vi "Threshold (subVI).vi"(8 "error in (no error)":errorcluster, 11 "Image  in":T1=refnum) -> (0 "error out":errorcluster, 2 "Cluster":cluster{sgl, "element":sgl}, 3 "Histogram":T2(graph))   [LabVIEW 2013]
uses:
  <vilib>/vision/Image Controls.llb/IMAQ Image.ctl
  <vilib>/vision/NI_Vision_Development_Module.lvlib
panel:
  out "brightened image":T1(plugin-control)
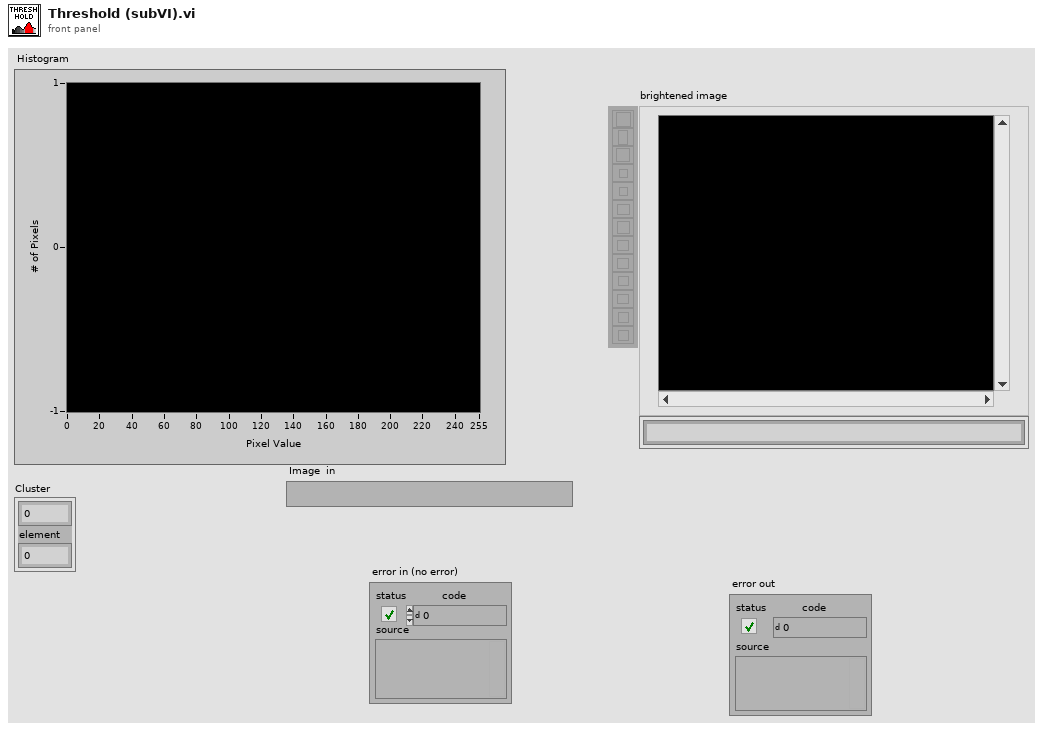
[diagram p1: front panel]
types:
  T1 = typedef "IMAQ Image.ctl" = refnum<image>
  T2 = cluster{"Starting Value":sgl, "Incremental Value":sgl, "Histogram":u32[]}
  T3 = typedef "Image Type" = u32
  T4 = cluster{"Brightness":sgl, "Contrast":sgl, "Gamma":sgl}
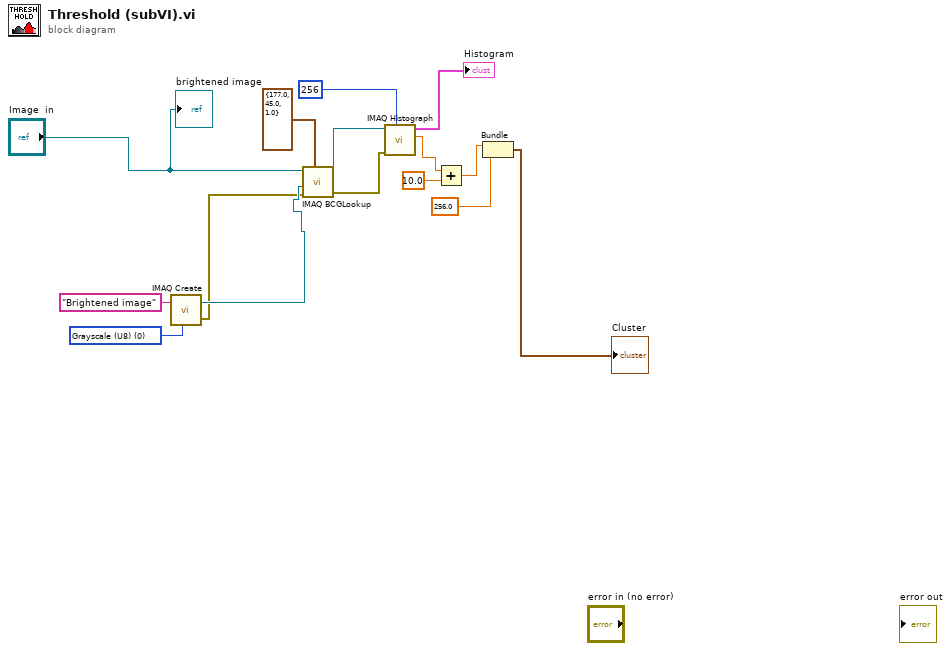
[diagram p0: block diagram]
diagram:
  w4 = T3 0 items=["Grayscale (U8)", "Grayscale (I16)", "Grayscale (SGL)", "Complex (CSG)", "RGB (U32)", "HSL (U32)", "RGB (U64)", "Grayscale (U16)"] ("Image Type")
  n1 = call "IMAQ Create"("Image Name"="Brightened image", "Image Type"=w4) -> ("New Image"=w2:T1, "error out"=w1:errorcluster)  [unwired: 3 in]
  n2 = call "IMAQ BCGLookup"("Image Src"="Image  in", "BCG Values"=T4 {"Brightness"=177.0, "Contrast"=45.0, "Gamma"=1.0}, "Image Dst"=w2, "error in (no error)"=w1) -> ("Image Dst Out"=w6:T1, "error out"=w10:errorcluster)  [unwired: 3 in]
  n3 = call "IMAQ Histograph"("Number of Classes"=256, "error in (no error)"=w10, "Image"=w6) -> ("Mean Value"=w12:sgl, "Histogram Graph"=→"Histogram":T2)  [unwired: 5 in, 2 out]
  n4 = Add(x=w12, y=sgl 10.0) -> (x+y=w14:sgl)
  n5 = Bundle(w14, "element"=sgl 256.0) -> (→"Cluster":cluster{sgl, "element":sgl})  [unwired: 1 in]
  "brightened image" <- "Image  in"
